vi "T7 Stream Read KAG-v2.vi"(0 "Connection ID In":refnum<k5>, 5 "IP Configuration":T1={"Connection ID In"=refnum, "Connection ID Out"=refnum, "Device IP"="192.168.126.147", "Port"=702}, 7 "Stream Configuration":T3={"Scan Rate (Hz)"=1000.0, "Samples Per Packet"=512, "Resolution Index"=0, "Buffer Size (bytes)"=32768, "NumScans"=1500, "Read Timeout (ms)"=5000.0, "Scan Table"=[{"Channel"=0, "BipGain"=0, "Input Config"="Single-Ended"}, {"Channel"=1, "BipGain"=0, "Input Config"="Single-Ended"}, {"Channel"=2, "BipGain"=0, "Input Config"="Single-Ended"}, {"Channel"=3, "BipGain"=0, "Input Config"="Single-Ended"}]} {"Samples Per Packet" max=512 step=1; "Buffer Size (bytes)" max=32768 step=1; "Resolution Index" max=8 step=1; "Scan Rate (Hz)" min=0.0 max=100000.0; "Scan Table"."BipGain" items=["x1", "x10", "x100", "x1000"]; "Scan Table"."Channel" step=1}, 9 "Secondary Stream Configurations":T2={"Settling Delay (*5 us)"=0.0, "Clock Source"=0, "Auto Target"=1} {"Auto Target" max=255 step=1; "Clock Source" max=2 step=2; "Settling Delay (*5 us)" min=0.0 max=5000.0 step=1.0}, 11 "error in":errorcluster) -> (6 "Read Array":u8[](array[numeric]) format="%.0x", 8 "TCP Data":string, 15 "error out":errorcluster)   [LabVIEW 2015]
doc: "Read Stream Data at Ethernet Socket 702."
uses:
  T7 Stream Config KAG.ctl
  T7 Secondary Configs KAG.ctl
  T7 IP Config KAG.ctl
  T7 Stream Globals KAG.vi
panel:
  in  "Tab Control":enum32{"TCP Read Data"}(tab)
  out "# of bytes received":i32
  out "# Bytes to Read":i32
  out "Scan Interval":dbl
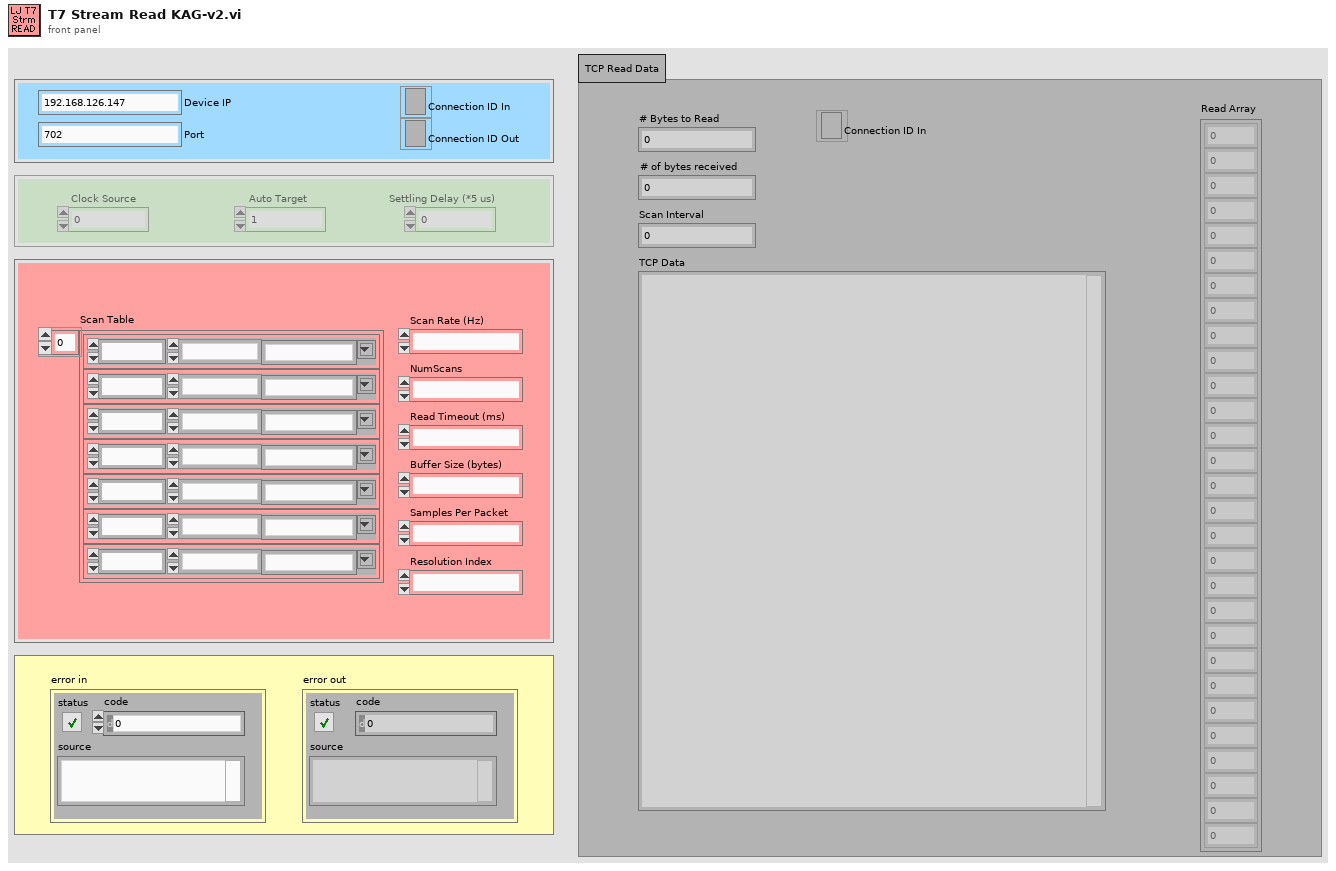
[diagram p1: front panel]
types:
  T1 = typedef "T7 IP Config KAG.ctl" = cluster{"Connection ID In":refnum<k5>, "Connection ID Out":refnum<k5>, "Device IP":string, "Port":i32}
  T2 = typedef "T7 Secondary Configs KAG.ctl" = cluster{"Settling Delay (*5 us)":dbl, "Clock Source":u32, "Auto Target":u32}
  T3 = typedef "T7 Stream Config KAG.ctl" = cluster{"Scan Rate (Hz)":dbl, "Samples Per Packet":u32, "Resolution Index":u32, "Buffer Size (bytes)":u32, "NumScans":u32, "Read Timeout (ms)":dbl, "Scan Table":cluster{"Channel":u32, "BipGain":u32, "Input Config":string}[]}
  T4 = cluster{"Channel":u32, "BipGain":u32, "Input Config":string}[]
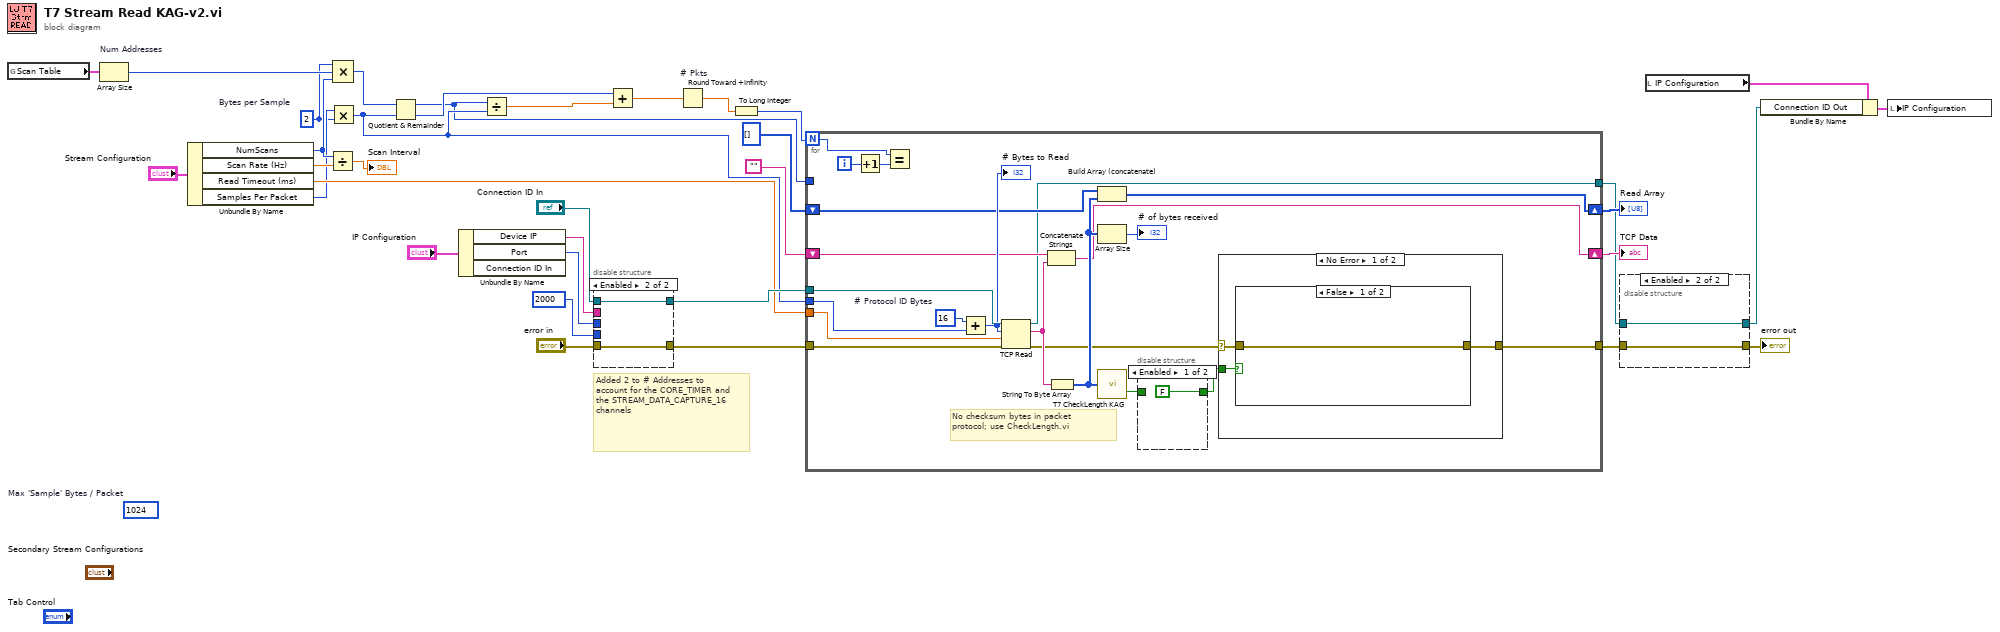
[diagram p0: block diagram]
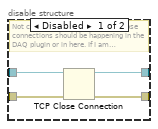
[diagram p2: hidden frame]
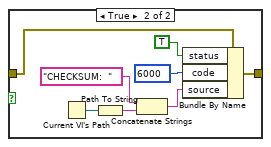
[diagram p4: hidden frame]
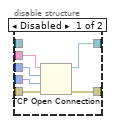
[diagram p6: hidden frame]
diagram:
  (unwired) 1024  # Max 'Sample' Bytes / Packet
  w9 = 2  # Bytes per Sample
  # "Added 2 to # Addresses to account for the CORE_TIMER and the STREAM_DATA_CAPTURE_16 channels"
  n1 = global read "T7 Stream Globals KAG.vi" "Scan Table"() -> (w28:T4)
  n2 = Array Size "Num Addresses"(array=w28) -> (size(s)=w21:i32)
  n3 = Unbundle By Name("Stream Configuration") -> ("NumScans"=w20:u32, "Scan Rate (Hz)"=w22:dbl, "Read Timeout (ms)"=w23:dbl, "Samples Per Packet"=w10:u32)
  n4 = Divide(x=w20, y=w22) -> (x/y=→"Scan Interval":dbl)
  n5 = Multiply(x=w10, y=w9) -> (x*y=w8:u32)
  n6 = Compound Arithmetic op=MULTIPLY(w9, w21, w20) -> (w18:u32)
  n7 = Quotient & Remainder(x=w18, y=w8) -> (x-y*floor(x/y)=w7:u32, floor(x/y)=w16:u32)
  n8 = Unbundle By Name("IP Configuration") -> ("Device IP"=w25:string, "Port"=w24:i32)  [unwired: 1 out]
  n9 = Divide(x=w7, y=w8) -> (x/y=w17:dbl)
  n10 = disable-structure shown="Enabled" {
    disable-tunnel: 2000 ("timeout ms (60000)") -> [w41 _]
    disable-tunnel: w25 -> [w40 _]
    disable-tunnel: "error in" -> [w39 w43]
    disable-tunnel: [w38 w43] -> w32
    disable-tunnel: [w37 w42] -> w31
    disable-tunnel: w24 -> [w36 _]
    disable-tunnel: "Connection ID In" -> [_ w42]
    frame Disabled {
      n11 = TCP Open Connection(address=w40, remote port or service name=w36, timeout ms (60000)=w41, error in (no error)=w39) -> (connection ID=w37:refnum<k5>, error out=w38:errorcluster)  [unwired: 1 out]
    }
    frame Enabled {
    }
  }
  n12 = Add(x=w16, y=w17) -> (x+y=w15:dbl)
  n13 = Round Toward +Infinity "# Pkts"(x=w15) -> (ceil(x): smallest int >= x=w14:dbl)
  n14 = To Long Integer(number=w14) -> (32bit integer=w13:i32)
  n15 = for {
    N: w13 -> [w47]
    tunnel: w32 -> [w63]
    tunnel: w31 -> [w62]
    tunnel: w23 -> [w57]
    tunnel: w8 -> [w49]
    shift-right: [w55] -> w30
    shift-left: u8[] [] ("unsigned byte array") -> [w54]
    shift-right: [w51] -> w35
    shift-left: "" -> [w53]
    tunnel: [w50] -> w2
    tunnel: w7 -> [_]
    tunnel: [w45] -> w4
    i -> [w48]
    w59 = u32 16  # # Protocol ID Bytes
    # "No checksum bytes in packet protocol; use CheckLength.vi"
    n16 = Increment(x=w48) -> (x+1=w46:i32)
    n17 = Equal?(x=w47, y=w46) -> ()  [unwired: 1 out]
    n18 = Add(x=w59, y=w49) -> (x+y=w58:u32)
    "# Bytes to Read" <- w58
    n19 = TCP Read(connection ID=w62, bytes to read=w58, error in (no error)=w63, 9:w57) -> (connection ID out=w45:refnum<k5>, data out=w52:string, error out=w44:errorcluster)  [unwired: 1 out]
    n20 = Concatenate Strings(w53, w52) -> (w51:string)
    n21 = String To Byte Array(string=w52) -> (unsigned byte array=w56:u8[])
    n22 = Build Array (concatenate)(w54, w56) -> (w55:u8[])
    n23 = Array Size(array=w56) -> (size(s)=→"# of bytes received":i32)
    n24 = call "T7 CheckLength KAG.vi"("Array"=w56) -> ("CheckLength Error"=w60:bool)  [unwired: 1 out]
    n25 = disable-structure shown="Enabled" {
      disable-tunnel: [FALSE w66] -> w61
      disable-tunnel: w60 -> [_ w66]
      frame Enabled {
      }
      frame Disabled {
      }
    }
    n26 = case shown="No Error" w44 {
      selector: w44 -> [w69 w79]
      tunnel: [w68 w79] -> w50
      tunnel: w61 -> [w67 _]
      frame No Error {
        n27 = case shown="False" w67 {
          tunnel: w69 -> [w70 w78]
          tunnel: [w70 w77] -> w68
          frame False {
          }
          frame True {
            n28 = Current VI's Path() -> (path=w75:path)
            n29 = Path To String(path=w75) -> (string=w73:string)
            n30 = Concatenate Strings("CHECKSUM:  " ("Substring"), w73) -> (w72:string)
            n31 = Bundle By Name(cluster=w78, "status"=TRUE, "code"=u32 6000 ("y"), "source"=w72) -> (w77:errorcluster)
          }
        }
      }
      frame Error {
      }
    }
  }
  "Read Array" <- w30
  "TCP Data" <- w35
  n32 = disable-structure shown="Enabled" {
    disable-tunnel: w4 -> [w83 w85]
    disable-tunnel: w2 -> [w82 w84]
    disable-tunnel: [w81 w85] -> w3
    disable-tunnel: [w80 w84] -> w1
    frame Disabled {
      # "Not clear whether the open and close connections should be happening in the DAQ plugin or in here. If I am recursively doing TCP reads, wouldn't make any sense to open and close tcp connection every time"
      n33 = TCP Close Connection(connection ID=w83, error in (no error)=w82) -> (connection ID out=w81:refnum<k5>, error out=w80:errorcluster)  [unwired: 1 in]
    }
    frame Enabled {
    }
  }
  "error out" <- w1
  n34 = local read "IP Configuration"() -> (w5:T1)
  n35 = Bundle By Name(cluster=w5, "Connection ID Out"=w3) -> (w6:T1)
  n36 = local write "IP Configuration"(w6) -> ()
